vi "test1.vi"() -> ()   [LabVIEW 2013]
uses:
  <vilib>/NI/Module Execution Interface/Engine Runtime/Execution States.ctl
  <vilib>/NI/TBM Modules/CVT Access/module/execution/CVT runtime.lvclass
  <vilib>/NI/TBM Modules/CVT Access/module/configuration/CVT configuration.lvclass
  Configuration/Standard Engine Configuration.lvclass
  Runtime/Standard Engine Runtime.lvclass
  <vilib>/NI/Tag Bus Module Framework/channel/channel classification.ctl
  <vilib>/NI/Tag Bus/tag/Data Type.ctl
  Configuration/Module Decimation.ctl
  Configuration/Module Error Configuration.ctl
  Configuration/Error Actions By Category.ctl
  <vilib>/NI/Tag Bus Module Framework/runtime/error classification.ctl
  Configuration/Error Actions.ctl
  Configuration/Supported Timing Sources.ctl
  Configuration/Standard Engine Configuration.lvclass/Standard Engine Configuration.ctl
  <vilib>/NI/Current Value Table/DataTypes/Double_Read.vi
  <vilib>/NI/Current Value Table/DataTypes/Double_Write.vi
  Configuration/Write Timing Source Type.vi
  <vilib>/NI/Current Value Table/Type to Enum.vi
  <vilib>/NI/Current Value Table/DataTypes/Double_Type To Enum.vi
  Configuration/Write Timing Source dt.vi
  Configuration/Find Module Specific Config.vi
  <vilib>/Utility/error.llb/Error Cluster From Error Code.vi
  <vilib>/NI/Current Value Table/FGVs/CVT Globals.vi
  <vilib>/NI/Current Value Table/FGVs/Tag Memory.vi
  <vilib>/NI/Current Value Table/Memory Block.vi
  <vilib>/NI/Current Value Table/DataTypes/Double_Memory Block.vi
  <vilib>/NI/Module Execution Interface/Engine Runtime/Engine Runtime Interface.lvclass
  <vilib>/NI/Current Value Table/Current Value Table.lvlib
  <vilib>/NI/Tag Bus Module Framework/channel/TBM channel.lvclass
  <vilib>/NI/Tag Bus/tag/tag descriptor.lvclass
  <vilib>/NI/Module Execution Interface/Engine Configuration/engine configuration.lvclass
  <vilib>/NI/Tag Bus Module Framework/runtime/TBM module execution interface.lvclass
panel:
  out "Engine State":T1=enum."Closed"
  in  "stop 2":bool
  out "error out 2":errorcluster
  out "error out":errorcluster
  out "B":dbl
  in  "A":dbl
  out "final error":errorcluster
  in  "stop":bool
  out "runtime error":errorcluster
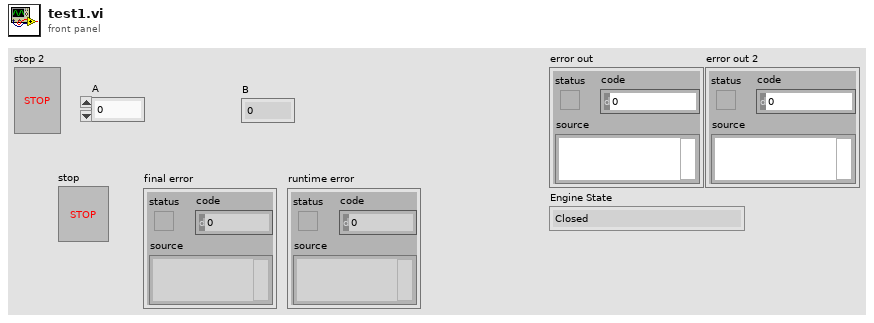
[diagram p1: front panel]
types:
  T1 = typedef "Engine Runtime Interface.lvclass/Execution States.ctl" = enum16{"Initializing", "Paused (Initialized)", "Running", "Set Safe Outputs", "Uninitializing", "Stopped (Uninitialized)", "Error (Uninitialized)", "Safe State (Uninitialized)", "Closed"}
  T2 = typedef "Standard Engine Configuration.lvclass/Supported Timing Sources.ctl" = enum16{"Use Module Timing Source", "1 kHz Clock", "1 MHz Clock", "Synchronize to Scan Engine"}
  T3 = typedef "Standard Engine Configuration.lvclass/Module Error Configuration.ctl" = cluster{"Module Error Configuration":T4[]}
  T4 = typedef "Standard Engine Configuration.lvclass/Error Actions By Category.ctl" = cluster{"error classification":T5, "Error Actions":T6[]}
  T5 = typedef "TBM module execution interface.lvclass/error classification.ctl" = enum16{"unknown", "none", "trivial", "recoverable", "critical"}
  T6 = typedef "Standard Engine Configuration.lvclass/Error Actions.ctl" = enum16{"Clear", "Notify", "Stop Component", "Stop Engine", "Safe State", "Attempt Recovery"}
  T7 = typedef "Standard Engine Configuration.lvclass/Module Decimation.ctl" = cluster{"Decimation":u16, "Offset":u16}
  T8 = typedef "tag bus.lvlib/tag descriptor.lvclass/Data Type.ctl" = enum16{"Double", "Single", "I64", "I32", "I16", "I8", "U64", "U32", "U16", "U8", "Boolean", "String", "Array of Double", "Array of Single", "Array of I64", "Array of I32", "Array of I16", "Array of I8", "Array of U64", "Array of U32", "Array of U16", "Array of U8", "Array of Boolean", "Array of String"}
  T9 = typedef "TBM channel.lvclass/channel classification.ctl" = enum16{"input data", "output data", "processing parameter", "processing result"}
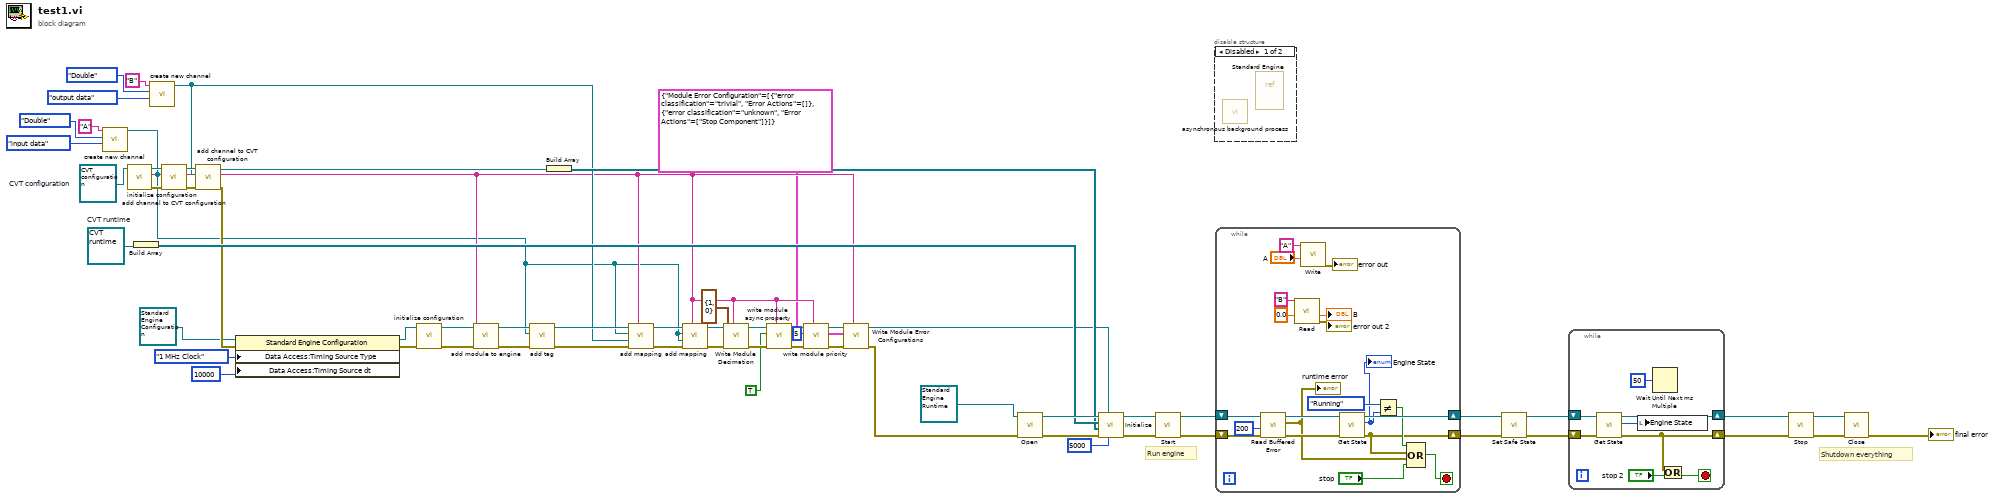
[diagram p0: block diagram]
diagram:
  w54 = refnum<class "CVT configuration.lvclass"> refnum  # CVT configuration
  w42 = refnum<class "CVT runtime.lvclass"> refnum  # CVT runtime
  # "Shutdown everything"
  # "Run engine"
  n1 = call <vilib>:"create new channel.vi"("channel classification"=channel_classification."input data", "data type"=Data_Type."Double", "channel name"="A") -> ("channel"=w12:refnum<class "TBM channel.lvclass">)  [unwired: 8 in]
  n2 = call-dynamic "initialize configuration.vi"("configuration in"=w54) -> ("error out"=w50:errorcluster, "instance identifier"=w17:string, "configuration out"=w51:refnum<class "CVT configuration.lvclass">)  [unwired: 8 in]
  n3 = Build Array(w42) -> (w40:refnum<class "CVT runtime.lvclass">[])
  n4 = call <vilib>:"create new channel.vi"("channel classification"=channel_classification."output data", "data type"=Data_Type."Double", "channel name"="B") -> ("channel"=w34:refnum<class "TBM channel.lvclass">)  [unwired: 8 in]
  n5 = call <vilib>:"add channel to CVT configuration.vi"("error in"=w50, "channel"=w12, "CVT configuration in"=w51) -> ("error out"=w52:errorcluster, "CVT configuration out"=w53:refnum<class "CVT configuration.lvclass">)  [unwired: 7 in]
  n6 = call <vilib>:"add channel to CVT configuration.vi"("error in"=w52, "channel"=w34, "CVT configuration in"=w53) -> ("error out"=w37:errorcluster, "CVT configuration out"=w43:refnum<class "CVT configuration.lvclass">)  [unwired: 7 in]
  n7 = property class="Standard Engine Configuration"(reference=refnum<class "Standard Engine Configuration.lvclass"> refnum ("Standard Engine Configuration"), error in=w37, "Data Access:Timing Source Type"=Supported_Timing_Sources."1 MHz Clock" ("Timing Source Type"), "Data Access:Timing Source dt"=u32 10000 ("Timing Source dt")) -> (reference out=w3:refnum<class "Standard Engine Configuration.lvclass">, error out=w5:errorcluster)
  n8 = call-dynamic "initialize configuration.vi"("error in"=w5, "configuration in"=w3) -> ("error out"=w30:errorcluster, "configuration out"=w29:refnum<class "Standard Engine Configuration.lvclass">)  [unwired: 7 in, 1 out]
  n9 = call-dynamic "add module to engine.vi"("error in"=w30, "module ID"=w17, "Standard Engine Configuration in"=w29) -> ("error out"=w32:errorcluster, "Standard Engine Configuration out"=w31:refnum<class "Standard Engine Configuration.lvclass">)  [unwired: 7 in]
  n10 = call <vilib>:"add tag.vi"("error in"=w32, "tag descriptor"=w12, "engine configuration in"=w31) -> ("error out"=w36:errorcluster, "engine configuration out"=w38:refnum<class "Standard Engine Configuration.lvclass">)  [unwired: 7 in]
  n11 = Build Array(w43) -> (w39:refnum<class "CVT configuration.lvclass">[])
  n12 = call <vilib>:"add mapping.vi"("owner ID"=w17, "error in"=w36, "channel"=w34, "tag descriptor"=w12, "engine configuration"=w38) -> ("error out"=w35:errorcluster, "engine configuration out"=w33:refnum<class "Standard Engine Configuration.lvclass">)  [unwired: 5 in]
  n13 = call <vilib>:"add mapping.vi"("owner ID"=w17, "error in"=w35, "channel"=w12, "tag descriptor"=w12, "engine configuration"=w33) -> ("error out"=w25:errorcluster, "engine configuration out"=w26:refnum<class "Standard Engine Configuration.lvclass">)  [unwired: 5 in]
  n14 = call "Write Module Decimation.vi"("Module ID"=w17, "error in"=w25, "Module Decimation"=T7 {"Decimation"=1, "Offset"=0}, "Standard Engine Repo Data in"=w26) -> ("error out"=w27:errorcluster, "Standard Engine Repo Data out"=w28:refnum<class "Standard Engine Configuration.lvclass">)  [unwired: 6 in]
  n15 = call "write module async property.vi"("Module ID"=w17, "error in"=w27, "async?"=TRUE, "Standard Engine Repo Data in"=w28) -> ("error out"=w21:errorcluster, "Standard Engine Repo Data out"=w19:refnum<class "Standard Engine Configuration.lvclass">)  [unwired: 6 in]
  n16 = call "write module priority.vi"("Module ID"=w17, "error in"=w21, "execution order priority"=5, "Standard Engine Repo Data in"=w19) -> ("error out"=w20:errorcluster, "Standard Engine Repo Data out"=w18:refnum<class "Standard Engine Configuration.lvclass">)  [unwired: 6 in]
  n17 = call "Write Module Error Configurations.vi"("Module ID"=w17, "error in"=w20, "Module Error Configuration"=T3 {"Module Error Configuration"=[{"error classification"=enum."trivial", "Error Actions"=[]}, {"error classification"=enum."unknown", "Error Actions"=[enum."Stop Component"]}]}, "Standard Engine Repo Data in"=w18) -> ("error out"=w24:errorcluster, "Standard Engine Repo Data out"=w23:refnum<class "Standard Engine Configuration.lvclass">)  [unwired: 6 in]
  n18 = call-dynamic "Open.vi"("error in"=w24, "Standard Engine in"=refnum<class "Standard Engine Runtime.lvclass"> refnum ("Standard Engine Runtime")) -> ("error out"=w57:errorcluster, "Standard Engine out"=w58:refnum<class "Standard Engine Runtime.lvclass">)  [unwired: 8 in]
  n19 = call-dynamic "Initialize.vi"("timeout in ms"=5000, "Engine Configuration"=w23, "error in"=w57, "Module Configurations"=w39, "Modules"=w40, "Standard Engine in"=w58) -> ("error out"=w56:errorcluster, "Standard Engine out"=w55:refnum<class "Standard Engine Runtime.lvclass">)  [unwired: 4 in]
  n20 = call-dynamic "Start.vi"("error in"=w56, "Standard Engine in"=w55) -> ("error out"=w60:errorcluster, "Standard Engine out"=w61:refnum<class "Standard Engine Runtime.lvclass">)  [unwired: 8 in]
  n21 = disable-structure shown="Disabled" {
    frame Disabled {
      n22 = call "asynchronous background process.vi"() -> ()  [unwired: 10 in, 2 out]
      n23 = vi-ref "Standard Engine.vi"() -> ()  [unwired: 1 out]
    }
    frame Enabled {
    }
  }
  n24 = while {
    shift-right: [w79] -> w7
    shift-left: w61 -> [w83]
    shift-right: [w73] -> w11
    shift-left: w60 -> [w82]
    stop <- w77 stop-if-true
    n25 = call-dynamic "Read Buffered Error.vi"("error in"=w82, "timeout in ms (0)"=200, "Standard Engine Runtime in"=w83) -> ("error out"=w80:errorcluster, "Engine Error"=w76:errorcluster, "Standard Engine Runtime out"=w81:refnum<class "Standard Engine Runtime.lvclass">)  [unwired: 6 in]
    "runtime error" <- w76
    n26 = call-poly <vilib>:"Read.vi"("Default"=0.0, "Tag Name"="B") -> ("error out"=→"error out 2":errorcluster, "Value"=→"B":dbl)  [unwired: 8 in]
    n27 = call-poly <vilib>:"Write.vi"("Value"="A", "Tag Name"="A") -> ("error out"=→"error out":errorcluster)  [unwired: 9 in]
    n28 = call-dynamic "Get State.vi"("error in"=w80, "Standard Engine Runtime in"=w81) -> ("error out"=w73:errorcluster, "Engine State"=w64:T1, "Standard Engine Runtime out"=w79:refnum<class "Standard Engine Runtime.lvclass">)  [unwired: 7 in]
    "Engine State" <- w64
    n29 = Not Equal?(x=Execution_States."Running" ("Engine State"), y=w64) -> (x != y?=w74:bool)
    n30 = Compound Arithmetic op=OR(w74, w73, w76, "stop") -> (w77:bool)
  }
  n31 = call-dynamic "Set Safe State.vi"("error in"=w11, "Standard Engine Runtime in"=w7) -> ("error out"=w8:errorcluster, "Standard Engine Runtime out"=w6:refnum<class "Standard Engine Runtime.lvclass">)  [unwired: 8 in]
  n32 = while {
    shift-right: [w89] -> w9
    shift-left: w6 -> [w90]
    shift-right: [w85] -> w10
    shift-left: w8 -> [w91]
    stop <- w86 stop-if-true
    n33 = call-dynamic "Get State.vi"("error in"=w91, "Standard Engine Runtime in"=w90) -> ("error out"=w85:errorcluster, "Engine State"=w84:T1, "Standard Engine Runtime out"=w89:refnum<class "Standard Engine Runtime.lvclass">)  [unwired: 7 in]
    n34 = local write "Engine State"(w84) -> ()
    n35 = Wait Until Next ms Multiple(millisecond multiple=u32 50) -> ()  [unwired: 1 out]
    n36 = Or(x=w85, y="stop 2") -> (x .or. y?=w86:bool)
  }
  n37 = call-dynamic "Stop.vi"("error in"=w10, "Standard Engine in"=w9) -> ("error out"=w62:errorcluster, "Standard Engine out"=w63:refnum<class "Standard Engine Runtime.lvclass">)  [unwired: 8 in]
  n38 = call-dynamic "Close.vi"("error in"=w62, "Standard Engine in"=w63) -> ("error out"=→"final error":errorcluster)  [unwired: 9 in]
